vi "stepinput_numarray.vi"(1 "Step Delay":i32(knob) scale=0.0..100.0, 2 "Samples":i32=128) -> (0 "OUTPUT ARRAY":dbl[](array[numeric]))   [LabVIEW 2009]
uses:
  <vilib>/Analysis/NI_AALBase.lvlib
panel:
  # "Assignment 5: Exercise 3_1 : Sub VI that generates a step input and outputs to a numeric array"
  # "A5_EX3_1_stepinput_numarray.vi"
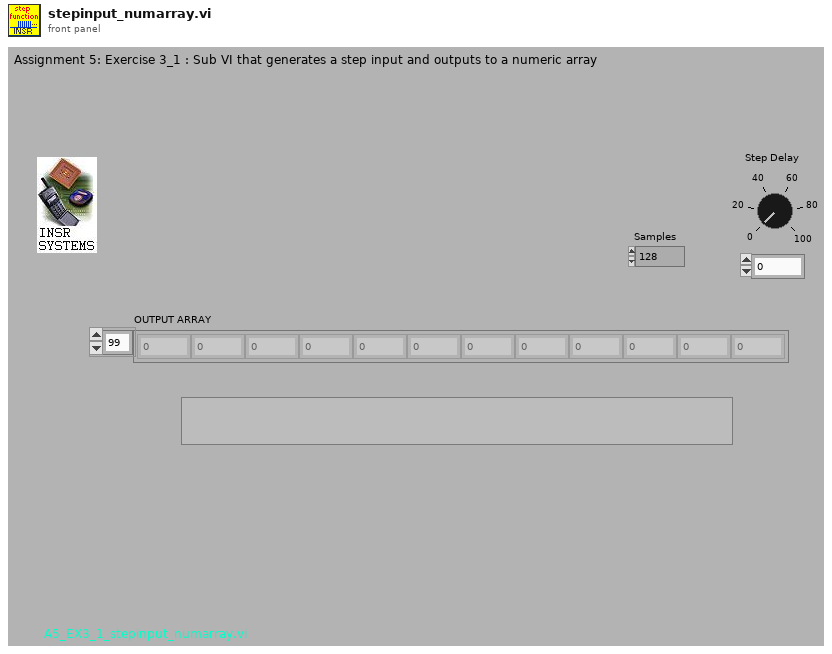
[diagram p1: front panel]
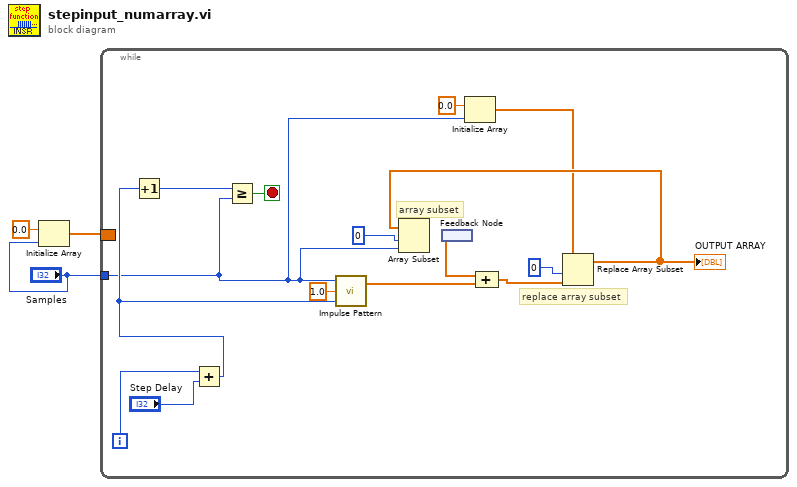
[diagram p0: block diagram]
diagram:
  n1 = Initialize Array(0.0 ("element"), "Samples") -> (w1:dbl[])
  n2 = while {
    tunnel: "Samples" -> [w4]
    border: w1 -> [_]
    i -> [w14]
    stop <- w19 stop-if-true
    # "array subset"
    # "replace array subset"
    n3 = Add(x=w14, y="Step Delay") -> (x+y=w13:i32)
    n4 = Increment(x=w13) -> (x+1=w7:i32)
    n5 = Greater Or Equal?(x=w7, y=w4) -> (x >= y?=w19:bool)
    n6 = call <vilib>:"Impulse Pattern.vi"("delay"=w13, "amplitude"=1.0, "samples"=w4) -> ("Impulse Pattern"=w11:dbl[])  [unwired: 1 out]
    n7 = feedback #1() -> (w16:dbl[])
    n8 = Initialize Array(0.0 ("element"), w4) -> (w5:dbl[])
    n9 = Compound Arithmetic op=ADD(w16, w11) -> (w10:dbl[])
    n10 = Replace Array Subset(array=w5, new element=w10, index=0) -> (w8:dbl[])
    "OUTPUT ARRAY" <- w8
    n11 = Array Subset(array=w8, index=0, length=w4) -> (w12:dbl[])
  }
